vi "Tracking.vi"() -> ()   [LabVIEW 2011]
panel:
  out "Motor Out":dbl
  out "Fire!":bool
  in  "Left Limit":bool
  in  "Right Limit":bool
  in  "Tolerance":dbl
  in  "Actual Position (x)":dbl
  in  "stop":bool
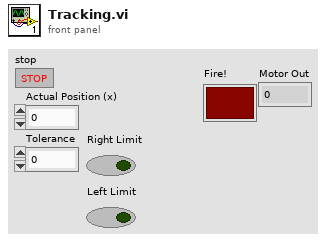
[diagram p1: front panel]
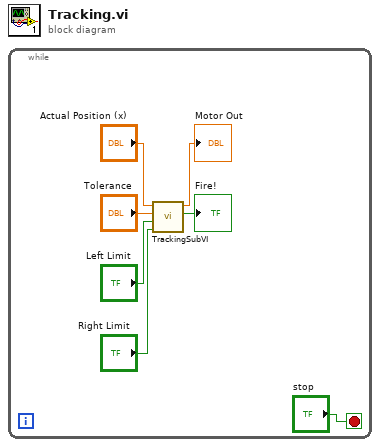
[diagram p0: block diagram]
diagram:
  n1 = while {
    stop <- "stop" stop-if-true
    n2 = call "TrackingSubVI.vi"("Right Limit"="Right Limit", "Left Limit"="Left Limit", "Tolerance"="Tolerance", "Actual Position (x)"="Actual Position (x)") -> ("Fire!"=→"Fire!":bool, "Motor Out"=→"Motor Out":dbl)  [unwired: 6 in]
  }
